vi "From String Array.vi"(8 "error in (no error)":errorcluster, 9 "String Array":string[](array[string]), 11 "Step Config in":refnum<class "Step Config.lvclass">) -> (0 "error out":errorcluster, 1 "Elements Left 2":string[](array[string]), 3 "Step Config out":refnum<class "Step Config.lvclass">)   [LabVIEW 2015, in "Step Config.lvclass"]
uses:
  Step Config.lvclass
  Step Config.lvclass/Step Config.ctl
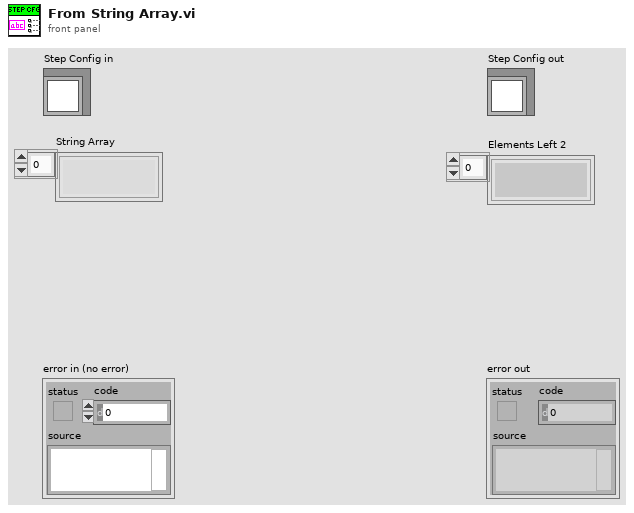
[diagram p1: front panel]
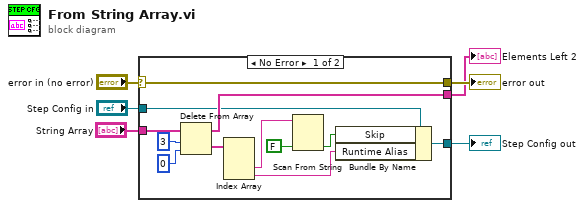
[diagram p0: block diagram]
diagram:
  n1 = case shown="No Error" "error in (no error)" {
    selector: "error in (no error)" -> [w18 w20]
    tunnel: [w18 w20] -> w5
    tunnel: [w11 w19] -> w3
    tunnel: "Step Config in" -> [w12 w19]
    tunnel: "String Array" -> [w17 _]
    tunnel: [w16 _] -> w1
    frame No Error {
      n2 = Delete From Array(array=w17, length=3, index=0) -> (deleted portion=w15:string[], array with subset deleted=w16:string[])
      n3 = Index Array(array=w15) -> (element #2=w8:string, element #3=w7:string)  [unwired: 3 in, 1 out]
      n4 = Scan From String(input string=w8, default 1=FALSE ("Skip")) -> (output 1=w9:bool)  [unwired: 3 in, 3 out]
      n5 = Bundle By Name(cluster=w12, "Skip"=w9, "Runtime Alias"=w7) -> (w11:refnum<class "Step Config.lvclass">)
    }
    frame Error {
    }
  }
  "error out" <- w5
  "Step Config out" <- w3
  "Elements Left 2" <- w1
